vi "sensor cmd flash block get.vi"(10 "block":u32, 11 "device_handle":u32) -> (1 "function return":i32, 2 "block out":u32, 3 "device_handle out":u32)   [LabVIEW 2019, in "apdm.lvlib"]
doc: "APDM_EXPORT int apdm_sensor_cmd_flash_block_get(apdm_device_handle_t device_handle, uint32_t *block);"
uses:
  apdm.lvlib
  Lee Lab/CP FES Walking 2018/Code/Working/LabVIEW/apdm.dll
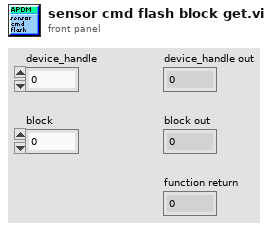
[diagram p1: front panel]
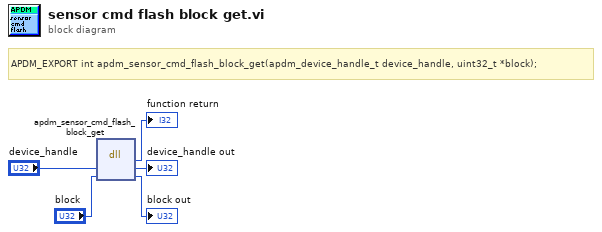
[diagram p0: block diagram]
diagram:
  # "APDM_EXPORT int apdm_sensor_cmd_flash_block_get(apdm_device_handle_t device_handle, uint32_t *block);"
  n1 = dll-call lib="C:/Users/jfalesi/Dropbox/Lee Lab/CP FES Walking 2018/Code/Working/LabVIEW/apdm.*" fn="apdm_sensor_cmd_flash_block_get"("device_handle"="device_handle", "block"="block") -> (→"function return":i32, "device_handle"=→"device_handle out":u32, "block"=→"block out":u32)  [unwired: 3 in, 2 out]
